vi "Begin.vi"(8 "error in":errorcluster) -> (0 "error out":errorcluster)   [LabVIEW 2017]
doc: "Called before other user functions, this VI is expected to open initial I/O refnums, load in file data, and do all program initialization. Notice that the <B>error out</B> terminal is simply used for data flow. Wiring it to other structures or subVIs ensures that this VI runs first."
uses:
  <vilib>/Rock Robotics/WPI/DriverStation/WPI_DriverStationRobotMode2.ctl
  SwerveLibrary/Swerve Motors.ctl
  SwerveLibrary/Drive Motors.ctl
  <vilib>/Rock Robotics/WPI/SafetyOutput/WPI_SafetyOutputConfigMenu.ctl
  Public/Documents/Cross The Road Electronics/Phoenix-LabVIEW/Motor Controller/Controls/CTRE_Phoenix_MotorControl_FeedbackDevice.ctl
  SwerveLibrary/Controllers.ctl
  <vilib>/Rock Robotics/WPI/Joystick/WPI_JoystickDeviceEnum.ctl
  SwerveLibrary/Sensors.ctl
  Robot Global Data.vi
  <vilib>/Rock Robotics/WPI/ThirdParty/Phoenix-LabVIEW/Pigeon IMU/CTRE_PigeonIMU_Open_CAN.vi
  Public/Documents/Cross The Road Electronics/Phoenix-LabVIEW/Pigeon IMU/CTRE_PigeonIMU_GetYPR.vi
  SwerveLibrary/Huskie Swerve.lvlib
panel:
  in  "PID gains":T1={"proportional gain (Kc)"=5.0, "integral time (Ti, min)"=0.032, "derivative time (Td, min)"=0.0} {"derivative time (Td, min)" format="%.3f"; "integral time (Ti, min)" format="%.8f"; "proportional gain (Kc)" format="%.8f"}
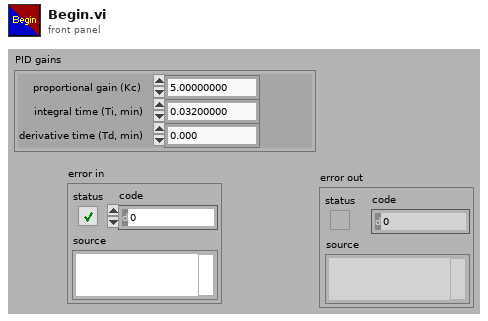
[diagram p1: front panel]
types:
  T1 = cluster{"proportional gain (Kc)":dbl, "integral time (Ti, min)":dbl, "derivative time (Td, min)":dbl}
  T2 = typedef "Huskie Swerve.lvlib/Drive Motors.ctl" = enum16{"Drive 1", "Drive 2", "Drive 3", "Drive 4"}
  T3 = typedef "Huskie Swerve.lvlib/Swerve Motors.ctl" = enum16{"Swerve 1", "Swerve 2", "Swerve 3", "Swerve 4"}
  T4 = typedef "WPI_DriverStationRobotMode2.ctl" = enum16{"Autonomous Disabled", "Autonomous Enabled", "Teleop Disabled", "Teleop Enabled", "Disconnected", "Finish", "Test Disabled", "Test Enabled", "Emergency Stopped"}
  T5 = typedef "WPI_SafetyOutputConfigMenu.ctl" = enum16{"Enable", "Disable"}
  T6 = typedef "CTRE_Phoenix_MotorControl_FeedbackDevice.ctl" = i8
  T7 = typedef "WPI_MotorControlDeviceRef.ctl" = cluster{"DeviceStatus":errorcluster, "Type":T8, "PWM":cluster{"PWM Channel":T9, "DeadBand":T10}, "CAN":cluster{"Device Number":u8, "SetOutput VI Ref":variant, "GetOutput VI Ref":variant, "Enable VI Ref":variant, "Disable VI Ref":variant, "Data":variant}, "Invert":bool, "DIO PWM":cluster{"PWM \"Enable\" Channel":T9, "DIOChannel":T11, "PWM Rate":dbl}}
  T8 = typedef "WPI_MotorControlType.ctl" = enum16{"PWM", "CAN", "DIO PWM"}
  T9 = typedef "FPGA_DIOPWMChannel.ctl" = enum8{"PWM 0", "PWM 1", "PWM 2", "PWM 3", "PWM 4", "PWM 5", "PWM 6", "PWM 7", "PWM 8", "PWM 9", "PWM MXP 0", "PWM MXP 1", "PWM MXP 2", "PWM MXP 3", "PWM MXP 4", "PWM MXP 5", "PWM MXP 6", "PWM MXP 7", "PWM MXP 8", "PWM MXP 9", "Invalid"}
  T10 = typedef "WPI_PWMDeadband.ctl" = cluster{"Name":string, "maxPositivePwm":i32, "minPositivePwm":i32, "centerPwm":i32, "maxNegativePwm":i32, "minNegativePwm":i32, "angularRange":u16}
  T11 = typedef "FPGA_DIOChannel.ctl" = enum8{"DIO 0", "DIO 1", "DIO 2", "DIO 3", "DIO 4", "DIO 5", "DIO 6", "DIO 7", "DIO 8", "DIO 9", "DIO MXP 0", "DIO MXP 1", "DIO MXP 2", "DIO MXP 3", "DIO MXP 4", "DIO MXP 5", "DIO MXP 6", "DIO MXP 7", "DIO MXP 8", "DIO MXP 9", "DIO MXP 10", "DIO MXP 11", "DIO MXP 12", "DIO MXP 13", "DIO MXP 14", "DIO MXP 15", "SPI Port CS1", "SPI Port CS2", "SPI Port CS3", "SPI Port MISO", "SPI Port MOSI", "Invalid"}
  T12 = typedef "WPI_JoystickDeviceEnum.ctl" = enum16{"USB 0", "USB 1", "USB 2", "USB 3", "USB 4", "USB 5"}
  T13 = typedef "Huskie Swerve.lvlib/Controllers.ctl" = enum16{"Joystick", "Buttons"}
  T14 = typedef "WPI_JoystickDevRef.ctl" = cluster{"Device":T12}
  T15 = typedef "Huskie Swerve.lvlib/Sensors.ctl" = enum16{"Gyro", "Vision USB", "Button Pressed", "Other sensor", "Generic Sensor"}
  T16 = typedef "CTRE_PigeonIMU_DeviceRef.ctl" = cluster{"DeviceStatus":errorcluster, "Device Number":u8, "Type":T17, "Device ID":u32, "Handle":u64, "UsageFrame":u32, "Library Path":path}
  T17 = typedef "CTRE_PigeonIMU_ConnectionType.ctl" = u32
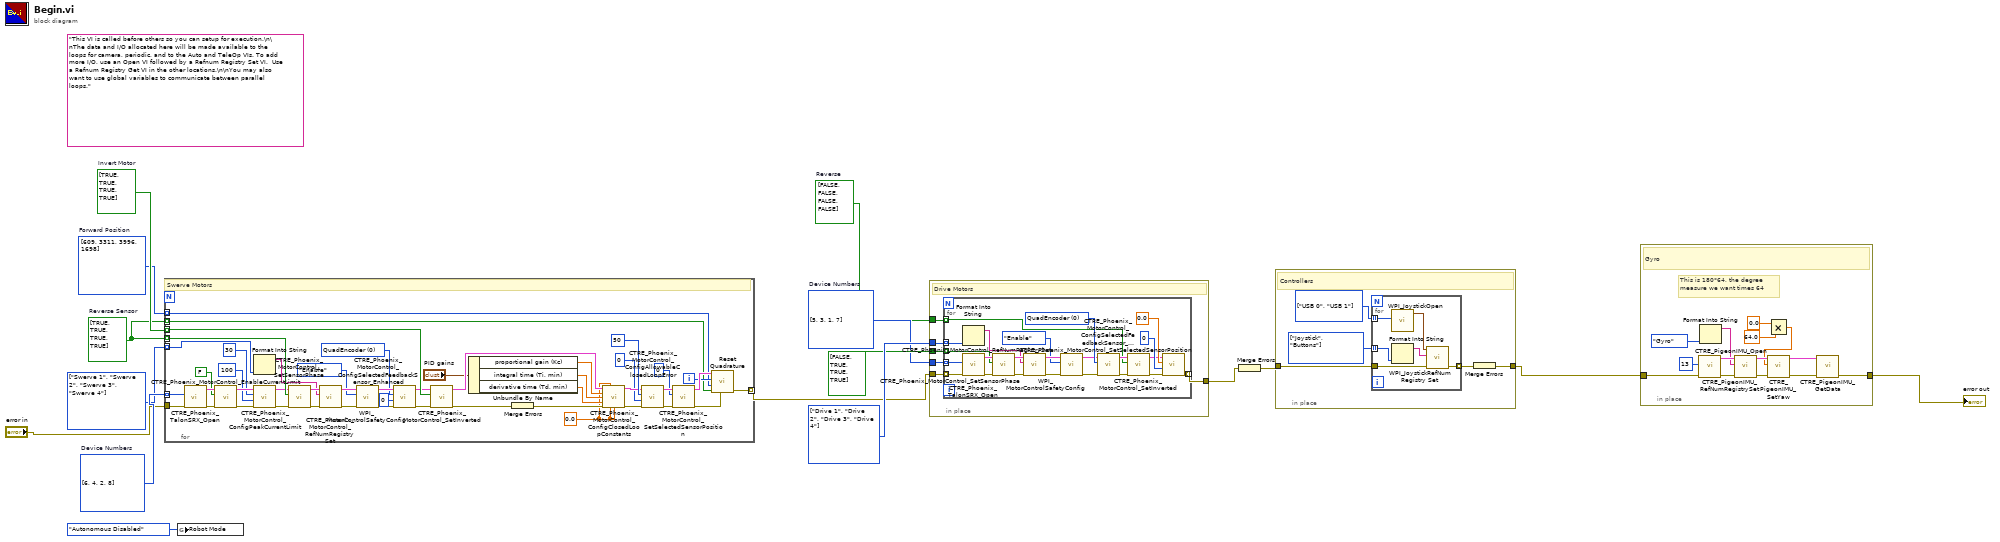
[diagram p0: block diagram]
diagram:
  w9 = T2[] [enum."Drive 1", enum."Drive 2", enum."Drive 3", enum."Drive 4"] items=["Drive 1", "Drive 2", "Drive 3", "Drive 4"] ("Array")
  w7 = i32[] [5, 3, 1, 7]  # Device Numbers
  w6 = bool[] [FALSE, FALSE, FALSE, FALSE]  # Reverse
  w13 = bool[] [TRUE, TRUE, TRUE, TRUE]  # Invert Motor
  w11 = bool[] [TRUE, TRUE, TRUE, TRUE]  # Reverse Sensor
  w15 = i32[] [6, 4, 2, 8]  # Device Numbers
  w12 = i32[] [609, 3311, 3996, 1698]  # Forward Position
  w14 = T3[] [enum."Swerve 1", enum."Swerve 2", enum."Swerve 3", enum."Swerve 4"] items=["Swerve 1", "Swerve 2", "Swerve 3", "Swerve 4"] ("Array")
  (unwired) "This VI is called before others so you can setup for execution.\n\nThe data and I/O allocated here will be made available to the loops for camera, periodic, and to the Auto and TeleOp VIs. To add more I/O, use an Open VI followed by a Refnum Registry Set VI.  Use a Refnum Registry Get VI in the other locations.\n\nYou may also want to use global variables to communicate between parallel loops."
  n1 = for {
    tunnel: w15 -> [w63] mode=indexing
    tunnel: w11 -> [w62] mode=indexing
    tunnel: w14 -> [w61] mode=indexing
    tunnel: w13 -> [w60] mode=indexing
    tunnel: w12 -> [w30] mode=indexing
    tunnel: w11 -> [w29] mode=indexing
    tunnel: "error in" -> [w28]
    tunnel: [w26] -> w5 mode=indexing
    i -> [w31]
    w19 = 0.0 ("F")
    w39 = T6 0 items=["None"=-1, "QuadEncoder"=0, "Analog"=2, "Tachometer"=4, "Pulse Width Encoded Position"=8, "Sensor Sum (S0 + S1)"=9, "Sensor Difference (D0 - D1)"=10, "Remote Source 0"=11, "Remote Source 1"=12, "Software Emulated"=15] ("Feedback Device")
    # "Swerve Motors"
    n2 = call "CTRE_Phoenix_TalonSRX_Open.vi"("error in"=w28, "Device Number"=w63) -> ("error out"=w47:errorcluster, "CAN Talon SRX Ref"=w56:T7)  [unwired: 8 in]
    n3 = call <vilib>:"CTRE_Phoenix_MotorControl_EnableCurrentLimit.vi"("error in (no error)"=w47, "Enable Current Limit?"=FALSE, "PhoenixMotorControlDevRef"=w56) -> ("error out"=w49:errorcluster, "PhoenixMotorControlDevRef"=w59:T7)  [unwired: 7 in]
    n4 = Format Into String(w61) -> (resulting string=w41:string)  [unwired: 3 in, 1 out]
    n5 = call <vilib>:"CTRE_Phoenix_MotorControl_ConfigPeakCurrentLimit.vi"("error in (no error)"=w49, "Peak Current Maximum Duration (ms)"=100, "Peak Current (Amps)"=30, "PhoenixMotorControlDevRef"=w59) -> ("error out"=w23:errorcluster, "PhoenixMotorControlDevRef"=w24:T7)  [unwired: 6 in]
    n6 = call "CTRE_Phoenix_MotorControl_SetSensorPhase.vi"("error in (no error)"=w23, "PhaseSensor"=w62, "PhoenixMotorControlDevRef"=w24) -> ("error out"=w52:errorcluster, "PhoenixMotorControlDevRef"=w55:T7)  [unwired: 7 in]
    n7 = call "CTRE_Phoenix_MotorControl_RefNumRegistrySet.vi"("error in (no error)"=w52, "refnum name"=w41, "PhoenixMotorControlDevRef"=w55) -> ("error out"=w51:errorcluster, "PhoenixMotorControlDevRef"=w54:T7)  [unwired: 7 in]
    n8 = call <vilib>:"WPI_MotorControlSafetyConfig.vi"("error in (no error)"=w51, "mode"=WPI_SafetyOutputConfigMenu."Enable", "MotorControlDevRef"=w54) -> ("error out"=w50:errorcluster, "MotorControlDevRef"=w53:T7)  [unwired: 7 in]
    n9 = call "CTRE_Phoenix_MotorControl_ConfigSelectedFeedbackSensor_Enhanced.vi"("error in (no error)"=w50, "pidLoopIdx"=0, "Feedback Device"=w39, "PhoenixMotorControlDevRef"=w53) -> ("error out"=w37:errorcluster, "PhoenixMotorControlDevRef"=w38:T7)  [unwired: 6 in]
    n10 = call "CTRE_Phoenix_MotorControl_SetInverted.vi"("error in (no error)"=w37, "Invert?"=w60, "PhoenixMotorControlDevRef"=w38) -> ("error out"=w35:errorcluster, "PhoenixMotorControlDevRef"=w33:T7)  [unwired: 7 in]
    n11 = Unbundle By Name("PID gains") -> ("proportional gain (Kc)"=w22:dbl, "integral time (Ti, min)"=w21:dbl, "derivative time (Td, min)"=w20:dbl)
    n12 = Merge Errors(w35) -> (w34:errorcluster)
    n13 = call "CTRE_Phoenix_MotorControl_ConfigClosedLoopConstants.vi"("PhoenixMotorControlDevRef"=w33, "slotIdx"=w19, "P"=w22, "I"=w21, "D"=w20, "error in (no error)"=w34, "F"=w19, "I Zone"=w19) -> ("PhoenixMotorControlDevRef"=w42:T7, "error out"=w45:errorcluster)  [unwired: 6 in]
    n14 = call <vilib>:"CTRE_Phoenix_MotorControl_ConfigAllowableClosedLoopError.vi"("error in (no error)"=w45, "slotIdx"=u32 0, "allowableClosedLoopError"=50, "PhoenixMotorControlDevRef"=w42) -> ("error out"=w44:errorcluster, "PhoenixMotorControlDevRef"=w43:T7)  [unwired: 6 in]
    n15 = call "CTRE_Phoenix_MotorControl_SetSelectedSensorPosition.vi"("error in (no error)"=w44, "New Sensor Position"=0, "PhoenixMotorControlDevRef"=w43) -> ("error out"=w27:errorcluster, "PhoenixMotorControlDevRef"=w32:T7)  [unwired: 7 in]
    n16 = call "Reset Quadrature.vi"("error in"=w27, "Reverse?"=w29, "Forward Position"=w30, "Module Number"=w31, "CAN Talon SRX Ref"=w32) -> ("error out"=w26:errorcluster)  [unwired: 5 in, 1 out]
  }
  n17 = global write "Robot Global Data.vi" "Robot Mode"(WPI_DriverStationRobotMode2."Autonomous Disabled" ("Robot Mode")) -> ()
  n18 = in-place {
    in-place-border: w9 -> [w69]
    in-place-border: bool[] [FALSE, TRUE, TRUE, TRUE] ("Reverse Feedback Sensor") -> [w68]
    in-place-border: w7 -> [w67]
    in-place-border: w6 -> [w66]
    in-place-border: w5 -> [w65]
    in-place-border: [w64] -> w4
    # "Drive Motors"
    n19 = for {
      tunnel: w69 -> [w92] mode=indexing
      tunnel: w68 -> [w87] mode=indexing
      tunnel: w67 -> [w91] mode=indexing
      tunnel: w66 -> [w70] mode=indexing
      tunnel: w65 -> [w90] mode=indexing
      tunnel: [w71] -> w64 mode=indexing
      w79 = T6 0 items=["None"=-1, "QuadEncoder"=0, "Analog"=2, "Tachometer"=4, "Pulse Width Encoded Position"=8, "Sensor Sum (S0 + S1)"=9, "Sensor Difference (D0 - D1)"=10, "Remote Source 0"=11, "Remote Source 1"=12, "Software Emulated"=15] ("Feedback Device")
      n20 = Format Into String(w92) -> (resulting string=w83:string)  [unwired: 3 in, 1 out]
      n21 = call "CTRE_Phoenix_TalonSRX_Open.vi"("error in"=w90, "Device Number"=w91) -> ("error out"=w88:errorcluster, "CAN Talon SRX Ref"=w89:T7)  [unwired: 8 in]
      n22 = call "CTRE_Phoenix_MotorControl_SetSensorPhase.vi"("error in (no error)"=w88, "PhaseSensor"=w87, "PhoenixMotorControlDevRef"=w89) -> ("error out"=w82:errorcluster, "PhoenixMotorControlDevRef"=w84:T7)  [unwired: 7 in]
      n23 = call "CTRE_Phoenix_MotorControl_RefNumRegistrySet.vi"("error in (no error)"=w82, "refnum name"=w83, "PhoenixMotorControlDevRef"=w84) -> ("error out"=w86:errorcluster, "PhoenixMotorControlDevRef"=w81:T7)  [unwired: 7 in]
      n24 = call <vilib>:"WPI_MotorControlSafetyConfig.vi"("error in (no error)"=w86, "mode"=WPI_SafetyOutputConfigMenu."Enable", "MotorControlDevRef"=w81) -> ("error out"=w85:errorcluster, "MotorControlDevRef"=w78:T7)  [unwired: 7 in]
      n25 = call "CTRE_Phoenix_MotorControl_ConfigSelectedFeedbackSensor_Enhanced.vi"("error in (no error)"=w85, "Feedback Device"=w79, "PhoenixMotorControlDevRef"=w78) -> ("error out"=w74:errorcluster, "PhoenixMotorControlDevRef"=w75:T7)  [unwired: 7 in]
      n26 = call "CTRE_Phoenix_MotorControl_SetInverted.vi"("error in (no error)"=w74, "Invert?"=w70, "PhoenixMotorControlDevRef"=w75) -> ("error out"=w73:errorcluster, "PhoenixMotorControlDevRef"=w72:T7)  [unwired: 7 in]
      n27 = call "CTRE_Phoenix_MotorControl_SetSelectedSensorPosition.vi"("error in (no error)"=w73, "pidLoopIdx"=u32 0, "New Sensor Position"=0.0, "PhoenixMotorControlDevRef"=w72) -> ("error out"=w71:errorcluster)  [unwired: 6 in, 1 out]
    }
  }
  n28 = Merge Errors(w4) -> (w3:errorcluster)
  n29 = in-place {
    in-place-border: w3 -> [w95]
    in-place-border: [w93] -> w2
    w96 = T12[] [enum."USB 0", enum."USB 1"] items=["USB 0", "USB 1", "USB 2", "USB 3", "USB 4", "USB 5"] ("Array")
    w97 = T13[] [enum."Joystick", enum."Buttons"] items=["Joystick", "Buttons"] ("Array")
    # "Controllers"
    n30 = for {
      tunnel: w97 -> [w103] mode=indexing
      tunnel: w96 -> [w102] mode=indexing
      tunnel: w95 -> [w99]
      tunnel: [w98] -> w94 mode=indexing
      n31 = call <vilib>:"WPI_JoystickOpen.vi"("JoystickDevice"=w102) -> ("JoystickDevRef"=w101:T14)  [unwired: 10 in]
      n32 = Format Into String(w103) -> (resulting string=w100:string)  [unwired: 3 in, 1 out]
      n33 = call <vilib>:"WPI_JoystickRefNum Registry Set.vi"("error in (no error)"=w99, "refnum name"=w100, "JoystickDevRef"=w101) -> ("error out"=w98:errorcluster)  [unwired: 7 in, 1 out]
    }
    n34 = Merge Errors(w94) -> (w93:errorcluster)
  }
  n35 = in-place {
    in-place-border: w2 -> [w109]
    in-place-border: [w108] -> w1
    # "This is 180*64, the degree\nmeasure we want times 64"
    # "Gyro"
    n36 = call-poly <vilib>:"CTRE_PigeonIMU_Open.vi"("error in"=w109, "Device Number"=u8 13) -> ("error out"=w117:errorcluster, "PigeonIMUDevRef"=w116:T16)  [unwired: 8 in]
    n37 = Format Into String(Sensors."Gyro" ("Enum")) -> (resulting string=w110:string)  [unwired: 3 in, 1 out]
    n38 = call <vilib>:"CTRE_PigeonIMU_RefNumRegistrySet.vi"("error in (no error)"=w117, "refnum name"=w110, "PigeonIMUDevRef"=w116) -> ("error out"=w115:errorcluster, "PigeonIMUDevRef"=w114:T16)  [unwired: 7 in]
    n39 = Multiply(x=0.0, y=64.0) -> (x*y=w104:dbl)
    n40 = call <vilib>:"CTRE_PigeonIMU_SetYaw.vi"("error in (no error)"=w115, "Value"=w104, "PigeonIMUDevRef"=w114) -> ("error out"=w112:errorcluster, "PigeonIMUDevRef"=w113:T16)  [unwired: 7 in]
    n41 = call-poly "CTRE_PigeonIMU_GetData.vi"("error in (no error)"=w112, "PigeonIMUDevRef"=w113) -> ("error out"=w108:errorcluster)  [unwired: 7 in, 2 out]
  }
  "error out" <- w1
